vi "Without Prefix.vi"(8 "error in (no error)":errorcluster, 11 "Test Case Test Double in":refnum<class "Test Case Test Double.lvclass">) -> (0 "error out":errorcluster, 3 "Test Case Test Double out":refnum<class "Test Case Test Double.lvclass">)   [LabVIEW 2020, in "Test Case Test Double.lvclass"]
uses:
  Test Case Test Double.lvclass
  C:/git/astemes-lunit/source/API/LUnit Test Case/LUnit Test Case.lvclass
  source/Core/LUnit Test Case/LUnit Test Case.lvclass/LUnit Test Case.ctl
  source/Core/LUnit Test Case/Private/Append Fail Result.vi
  source/Core/LUnit Test Case/Private/Append Pass Result.vi
  source/Core/LUnit Test Case/Private/Run In UI.vi
  <vilib>/Utility/error.llb/Clear Errors.vi
  source/Core/LUnit Test Case/LUnit Test Case.lvclass
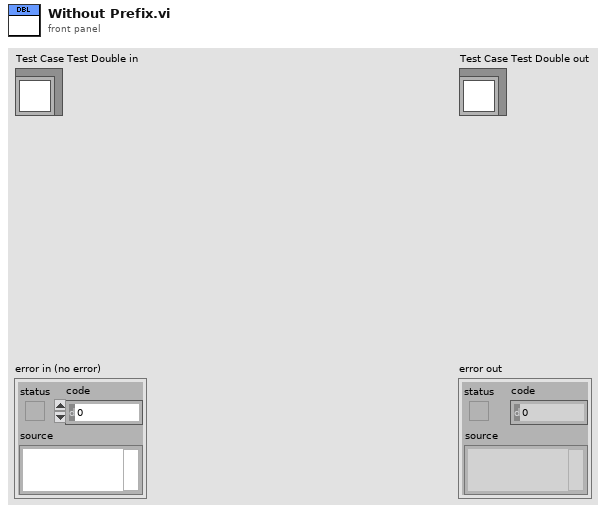
[diagram p1: front panel]
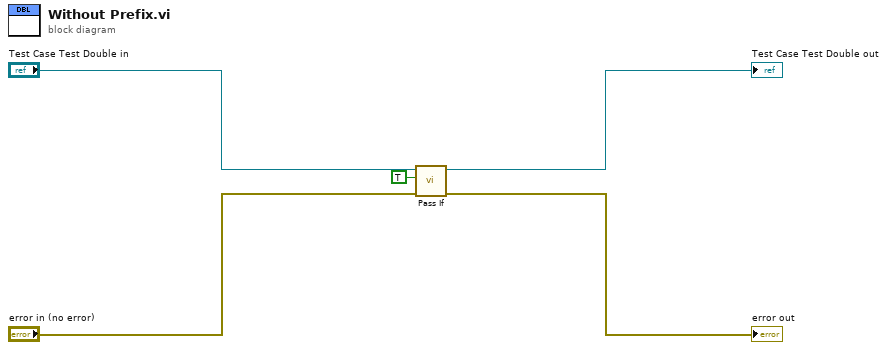
[diagram p0: block diagram]
diagram:
  n1 = call "Pass If.vi"("error in (no error)"="error in (no error)", "Pass?"=TRUE, "LUnit Test Case In"="Test Case Test Double in") -> ("error out"=→"error out":errorcluster, "LUnit Test Case Out"=→"Test Case Test Double out":refnum<class "Test Case Test Double.lvclass">)  [unwired: 7 in]
